vi "Read Window Position and Size.vi"(8 "error in":errorcluster) -> (0 "error out":errorcluster, 3 "Bounds":T1)   [LabVIEW 2019, in "Panther Dashboard.lvlib"]
uses:
  Panther Dashboard.lvlib
  <vilib>/Utility/miscctls.llb/LVRectTypeDef.ctl
  <vilib>/Utility/config.llb/Read Key (String).vi
  <vilib>/Utility/config.llb/NI_LVConfig.lvlib
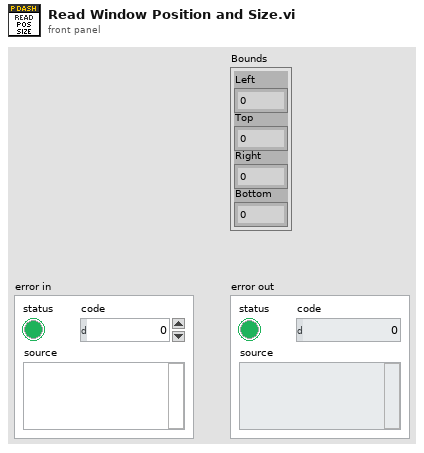
[diagram p1: front panel]
types:
  T1 = typedef "LVRectTypeDef.ctl" = cluster{"Left":i16, "Top":i16, "Right":i16, "Bottom":i16}
  T2 = typedef "NI_LVConfig.lvlib/Config Data RefNum.ctl" = refnum<k1>
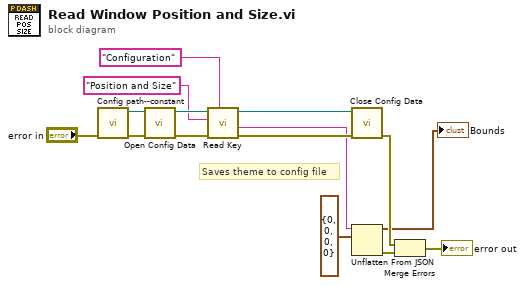
[diagram p0: block diagram]
diagram:
  # "Saves theme to config file"
  n1 = call "Config path--constant.vi"("error in (no error)"="error in") -> ("error out"=w13:errorcluster, "Config Path"=w4:path)  [unwired: 9 in]
  n2 = call <vilib>:"Open Config Data.vi"("error in (no error)"=w13, "configuration file path"=w4) -> ("error out"=w14:errorcluster, "refnum"=w7:T2)  [unwired: 7 in, 1 out]
  n3 = call-poly <vilib>:"Read Key.vi"("section"="Configuration", "error in (no error)"=w14, "key"="Position and Size", "refnum"=w7) -> ("error out"=w9:errorcluster, "value"=w1:string, "refnum out"=w8:T2)  [unwired: 4 in, 1 out]
  n4 = call <vilib>:"Close Config Data.vi"("error in (no error)"=w9, "refnum"=w8) -> ("error out"=w15:errorcluster)  [unwired: 8 in, 1 out]
  n5 = Unflatten From JSON(JSON string=w1, type and defaults=T1 {"Left"=0, "Top"=0, "Right"=0, "Bottom"=0} ("NewBnds")) -> (value=→"Bounds":T1, error out=w10:errorcluster)  [unwired: 5 in]
  n6 = Merge Errors(w15, w10) -> (→"error out":errorcluster)
